vi "Delete Project Destination on Error.vi"(11 "Project Destination Root":path) -> ()   [LabVIEW 2016]
panel:
  out "error out":errorcluster
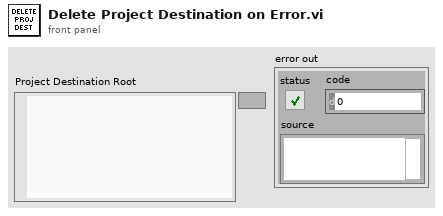
[diagram p1: front panel]
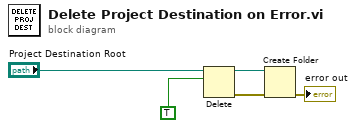
[diagram p0: block diagram]
diagram:
  n1 = Delete(path (use dialog)="Project Destination Root", entire hierarchy (F)=TRUE) -> (deleted path=w3:path, error out=w2:errorcluster)  [unwired: 3 in, 1 out]
  n2 = Create Folder(path (use dialog)=w3, error in=w2) -> (error out=→"error out":errorcluster)  [unwired: 1 in, 2 out]
